vi "Get Measure.vi"(8 "error in (no error)":errorcluster caption="entrée d'erreur (pas d'erreur)", 11 "Class Spectrum_Analyser RS306B en entrée":refnum<class "Class Spectrum_Analyser RS306B.lvclass">) -> (0 "error out":errorcluster caption="sortie d'erreur", 3 "Class Spectrum_Analyser RS306B en sortie":refnum<class "Class Spectrum_Analyser RS306B.lvclass">)   [LabVIEW 2020, in "Library Instrument & Equipement.lvlib" / "Library Spectrum Analyser.lvlib" / "Class Spectrum_Analyser RS306B.lvclass"]
uses:
  Class Spectrum_Analyser RS306B.lvclass
  C:/Users/ngarcin/OneDrive - Altyor/Standard TB/Class/Spectrum Analyser/Class Spectrum Analyser (Default)/Class Spectrum Analyser (Default).lvclass
  Commun VI/TypeDef/Liste Error.ctl
  Class Spectrum_Analyser RS306B.lvclass/Class Spectrum_Analyser RS306B.ctl
  Commun VI/Library Commun.lvlib
  Library Spectrum Analyser.lvlib
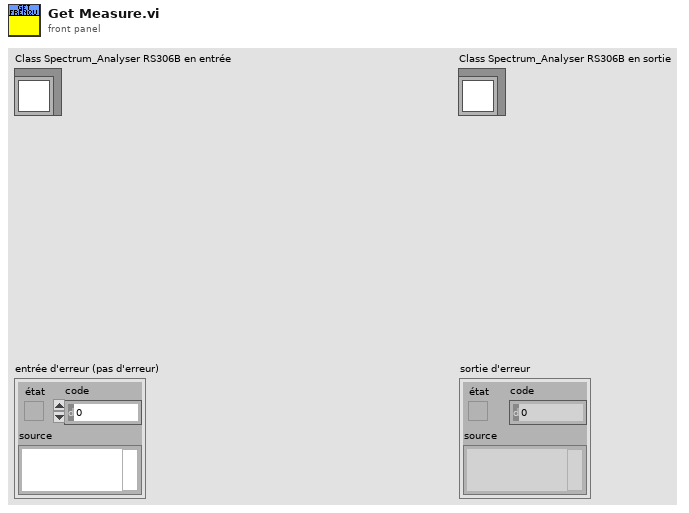
[diagram p1: front panel]
types:
  T1 = enum16{"CENTER FREQUENCY", "FREQUENCY SPAN", "RESOLUTION BW", "MAX REAL TIME SPAN (SET)", "START FREQUENCY", "STOP FREQUENCY", "FREQ STEP SIZE", "AUTO FREQ STEP ON", "AUTO FREQ STEP OFF", "AUTO RES BW ON", "AUTO RES BW OFF", "FFT WINDOW TYPE", "# POINTS", "RBW PROCESS ON", "RBW PROCESS OFF", "GAIN/BW OPTIMIZATION"}
  T2 = enum16{"RUN ACQUISITION  & GET RESULT", "GET LAST ACQUISITION RESULT"}
  T3 = typedef "Library Commun.lvlib/Liste Error.ctl" = enum16{"Firebase Driver - Get Document", "Firebase Driver - Get Document With Where", "Firebase Driver - Delete Document", "Firebase Driver - Set Document", "Firebase Driver - Update Document", "Firebase Altyor - Search Document Bench", "Firebase Altyor - Class Not in Firebase", "Spectrum_Analyser - Timeout", "Relay Board - Qty Relay", "DIO - Pb Funtion", "Power_Supply - Peripherical not find", "Mutimeter - Peripherical not find", "Instrument - Function Not Used", "Instrument - Instrument name not specified", "Instrument - Allready Initialised", "Instrument - TimeOut", "Instrument - the instrument must be Initialise before", "Instrument - Frame Not received", "Instrument - Frame Nok", "Test - Initialise the File_for_Save", "Test - Timeout", "Test - Cmd Error", "FGV - Variable ", "BDD FireBase - Define Class", "SN - Class Not Define"}
  T4 = enum16{"PRESET (SET)", "OPERATION CONDITION (READ)", "OPERATION ENABLE", "OPERATION EVENT (READ)", "OPERATION PTRANSITION", "OPERATION NTRANSITION", "QUESTIONABLE CONDITION (READ)", "QUESTIONABLE ENABLE", "QUESTIONABLE EVENT (READ)", "QUESTIONABLE PTRANSITION", "QUESTIONABLE NTRANSITION", "QUESTIONABLE FREQ CONDITION (READ)", "QUESTIONABLE FREQ ENABLE", "QUESTIONABLE FREQ EVENT (READ)", "QUESTIONABLE FREQ PTRANSITION", "QUESTIONABLE FREQ NTRANSITION", "QUESTIONABLE INTEGRITY CONDITION (READ)", "QUESTIONABLE INTEGRITY ENABLE", "QUESTIONABLE INTEGRITY EVENT (READ)", "QUESTIONABLE INTEGRITY PTRANSITION", "QUESTIONABLE INTEGRITY NTRANSITION", "QUESTIONABLE CALIB CONDITION (READ)", "QUESTIONABLE CALIB ENABLE", "QUESTIONABLE CALIB EVENT (READ)", "QUESTIONABLE CALIB PTRANSITON", "QUESTIONABLE CALIB NTRANSITION", "QUESTIONABLE POWER CONDITION (READ)", "QUESTIONABLE POWER ENABLE", "QUESTIONABLE POWER EVENT (READ)", "QUESTIONABLE POWER PTRANSITION", "QUESTIONABLE POWER NTRANSITION", "QUESTIONABLE TEMP CONDITION (READ)", "QUESTIONABLE TEMP ENABLE", "QUESTIONABLE TEMP EVENT (READ)", "QUESTIONABLE TEMP PTRANSITION", "QUESTIONABLE TEMP NTRANSITION"}
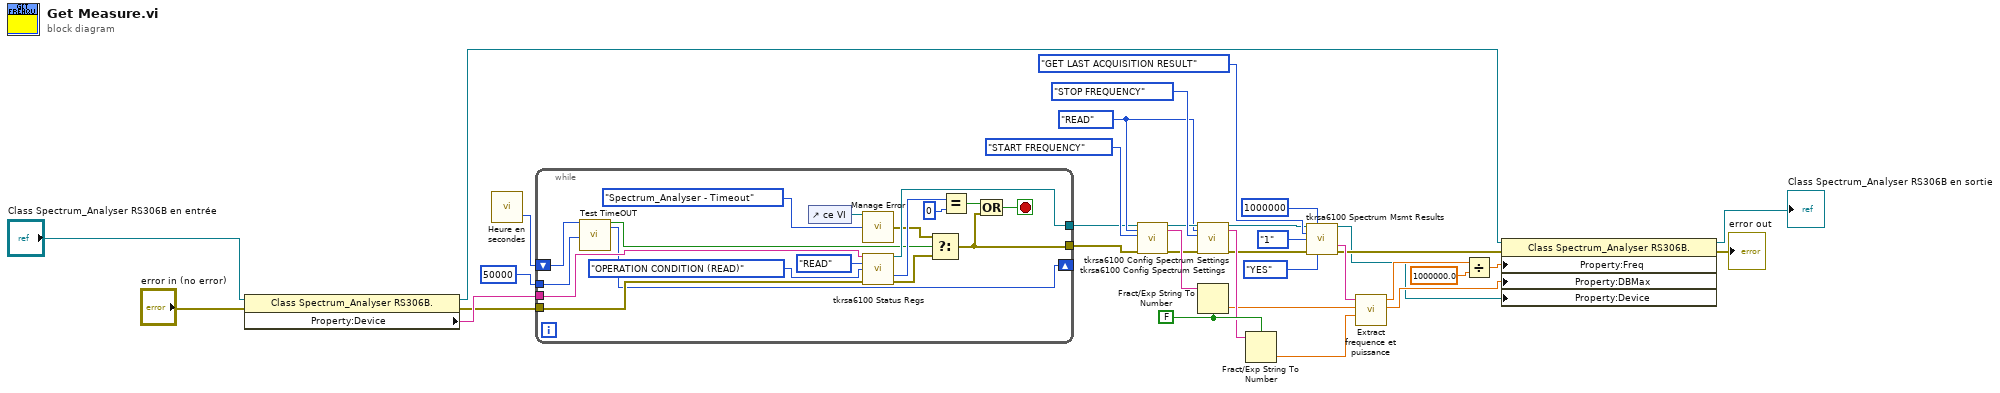
[diagram p0: block diagram]
diagram:
  w24 = FALSE ("utiliser le séparateur décimal du système (V)")
  w19 = enum16{"SET", "READ"}."READ" ("Set/Read\nSpectrum Setting (SET)")
  n1 = property class="Class Spectrum_Analyser RS306B."(reference="Class Spectrum_Analyser RS306B en entrée", error in="error in (no error)") -> (reference out=w28:refnum<class "Class Spectrum_Analyser RS306B.lvclass">, error out=w31:errorcluster, "Property:Device"=w33:string)
  n2 = call "Heure en secondes.vi"() -> ("Heure en milisecondes"=w27:u32)  [unwired: 2 in, 1 out]
  n3 = while {
    tunnel: w31 -> [w52]
    tunnel: [w51] -> w3
    tunnel: [w35] -> w7
    tunnel: w33 -> [w46]
    tunnel: u32 50000 ("Timeout") -> [w45]
    shift-right: [w43] -> _
    shift-left: w27 -> [w44]
    stop <- w41 stop-if-true
    n4 = call "Test TimeOUT.vi"("OLD Time"=w44, "TimeOut ms"=w45) -> ("Timeout ?"=w38:bool, "NEW Time"=w43:u32)  [unwired: 13 in, 3 out]
    n5 = control-ref of="ce VI"() -> (w40:refnum<vi>)
    n6 = call "Manage Error.vi"("VI in Error"=w40, "Code Erreur"=Liste_Error."Spectrum_Analyser - Timeout") -> ("error out"=w37:errorcluster)  [unwired: 13 in]
    n7 = call "tkrsa6100 Status Regs.vi"("VISA Resource Name"=w46, "Set/Read\nStatus Register (SET)"=enum16{"SET", "READ"}."READ" ("Set/Read\nStatus Register (SET)"), "Register (PRESET)"=T4."OPERATION CONDITION (READ)", "error in (no error)"=w52) -> ("dup VISA Resource Name"=w51:refnum<visa-resource-name>, "Register #"=w48:i32, "error out"=w36:errorcluster)  [unwired: 7 in, 2 out]
    n8 = Select(t=w37, s=w38, f=w36) -> (s? t:f=w35:errorcluster)
    n9 = Equal?(x=w48, y=u32 0) -> (x = y?=w42:bool)
    n10 = Compound Arithmetic op=OR ("Opérateur arithmétique")(w42, w35) -> (w41:bool)
  }
  n11 = call "tkrsa6100 Config Spectrum Settings.vi"("VISA Resource Name"=w3, "Set/Read\nSpectrum Setting (SET)"=w19, "Spectrum Settings\n (CENTER FREQUENCY)"=T1."START FREQUENCY" ("Spectrum Settings\n (CENTER FREQUENCY)"), "error in (no error)"=w7) -> ("dup VISA Resource Name"=w20:refnum<visa-resource-name>, "Spectrum Setting\nResponse String"=w22:string, "error out"=w18:errorcluster)  [unwired: 13 in]
  n12 = call "tkrsa6100 Config Spectrum Settings.vi"("VISA Resource Name"=w20, "Set/Read\nSpectrum Setting (SET)"=w19, "Spectrum Settings\n (CENTER FREQUENCY)"=T1."STOP FREQUENCY" ("Spectrum Settings\n (CENTER FREQUENCY)"), "error in (no error)"=w18) -> ("dup VISA Resource Name"=w8:refnum<visa-resource-name>, "Spectrum Setting\nResponse String"=w23:string, "error out"=w9:errorcluster)  [unwired: 13 in]
  n13 = Fract/Exp String To Number(use system decimal point (T)=w24, string=w22) -> (number=w15:dbl)  [unwired: 2 in, 1 out]
  n14 = Fract/Exp String To Number(use system decimal point (T)=w24, string=w23) -> (number=w16:dbl)  [unwired: 2 in, 1 out]
  n15 = call "tkrsa6100 Spectrum Msmt Results.vi"("VISA Resource Name"=w8, "Byte Count\n(100000)"=1000000 ("Byte Count\n(100000)"), "Run Acquisition and/or \nGet Result (RUN ACQUISITION & GET RESULT)"=T2."GET LAST ACQUISITION RESULT" ("Run Acquisition and/or \nGet Result (RUN ACQUISITION & GET RESULT)"), "Spectrum Trace(1)"=enum16{"1", "2", "3", "MATH", "SGRAM"}."1", "error in (no error)"=w9, "Convert Resp\nString(NO)"=enum16{"NO", "YES"}."YES" ("Convert Resp\nString(NO)")) -> ("dup VISA Resource Name"=w2:refnum<visa-resource-name>, "Converted Sgl Float\nResponse String"=w14:string, "error out"=w4:errorcluster)  [unwired: 5 in, 2 out]
  n16 = call "Extract frequence et puissance.vi"("Frequence Stop"=w16, "Frequence Start"=w15, "Reception RSA306"=w14) -> ("DBMax"=w5:dbl, "Freq"=w25:dbl)  [unwired: 7 in]
  n17 = Divide(x=w25, y=1000000.0 ("x")) -> (x/y=w6:dbl)
  n18 = property class="Class Spectrum_Analyser RS306B."(reference=w28, error in=w4, "Property:Freq"=w6, "Property:DBMax"=w5, "Property:Device"=w2) -> (reference out=→"Class Spectrum_Analyser RS306B en sortie":refnum<class "Class Spectrum_Analyser RS306B.lvclass">, error out=→"error out":errorcluster)
